vi "Test Factory.vi"() -> ()   [LabVIEW 2013]
uses:
  source/Control Packets/ControlPacket/ControlPacket.lvclass
panel:
  out "Array":refnum<class "ControlPacket.lvclass">[](array[class])
  out "Remaining Packets":u8[](array[numeric]) format="%08b"
  in  "stop":bool
  out "error out":errorcluster
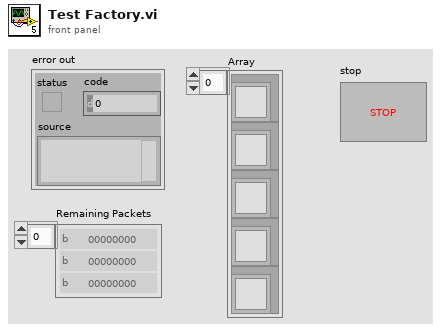
[diagram p1: front panel]
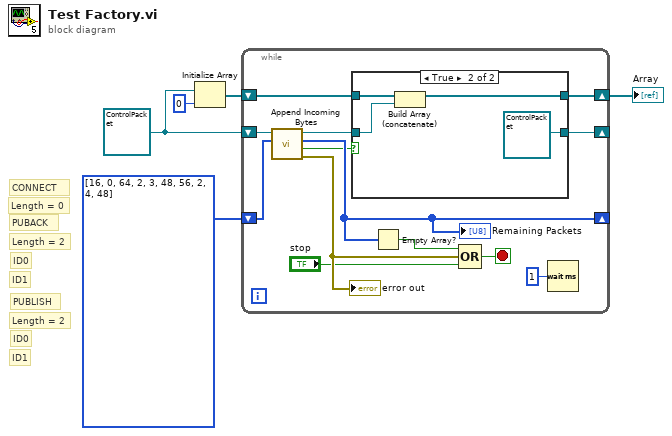
[diagram p0: block diagram]
diagram:
  w3 = refnum<class "ControlPacket.lvclass"> refnum ("ControlPacket.lvclass")
  # "ID1"
  # "ID0"
  # "Length = 2"
  # "PUBLISH"
  # "ID1"
  # "ID0"
  # "Length = 2"
  # "PUBACK"
  # "Length = 0"
  # "CONNECT"
  n1 = Initialize Array(w3, 0 ("dimension size")) -> (w4:refnum<class "ControlPacket.lvclass">[])
  n2 = while {
    shift-right: [w17] -> _
    shift-left: w3 -> [w18]
    shift-right: [w8] -> _
    shift-left: u8[] [16, 0, 64, 2, 3, 48, 56, 2, 4, 48] ("Incoming Packets") -> [w6]
    shift-right: [w9] -> w1
    shift-left: w4 -> [w11]
    stop <- w14 stop-if-true
    n3 = call "Append Incoming Bytes.vi"("Incoming Packets"=w6, "Incomplete ControlPacket"=w18) -> ("error out"=w15:errorcluster, "Complete Packet"=w7:bool, "Remaining Packets"=w8:u8[], "ControlPacket"=w16:refnum<class "ControlPacket.lvclass">)  [unwired: 6 in]
    "error out" <- w15
    "Remaining Packets" <- w8
    n4 = case shown="True" w7 {
      tunnel: [w20 refnum<class "ControlPacket.lvclass"> refnum ("ControlPacket.lvclass")] -> w17
      tunnel: w16 -> [w20 w22]
      tunnel: w11 -> [w19 w23]
      tunnel: [w19 w21] -> w9
      frame False {
      }
      frame True {
        n5 = Build Array (concatenate)(w23, w22) -> (w21:refnum<class "ControlPacket.lvclass">[])
      }
    }
    n6 = Empty Array?(array=w8) -> (empty?=w10:bool)
    n7 = Compound Arithmetic op=OR(w10, w15, "stop") -> (w14:bool)
    n8 = Wait (ms)(milliseconds to wait=u32 1) -> ()  [unwired: 1 out]
  }
  "Array" <- w1
